vi "Process Laser State.vi"(7 "error in (no error)":errorcluster, 9 "Data":string, 10 "object in":refnum<class "Laser Ethernet Cabinet.lvclass">) -> (0 "error out":errorcluster, 3 "object out":refnum<class "Laser Ethernet Cabinet.lvclass">)   [LabVIEW 2023, in "Laser Ethernet Cabinet.lvclass"]
uses:
  Laser Ethernet Cabinet.lvclass
  raw_status.ctl
  Laser Ethernet Cabinet.lvclass/Laser Ethernet Cabinet.ctl
  <vilib>/Utility/Data Type/NI_Data Type.lvlib
panel:
  in  "Raw Status":T1
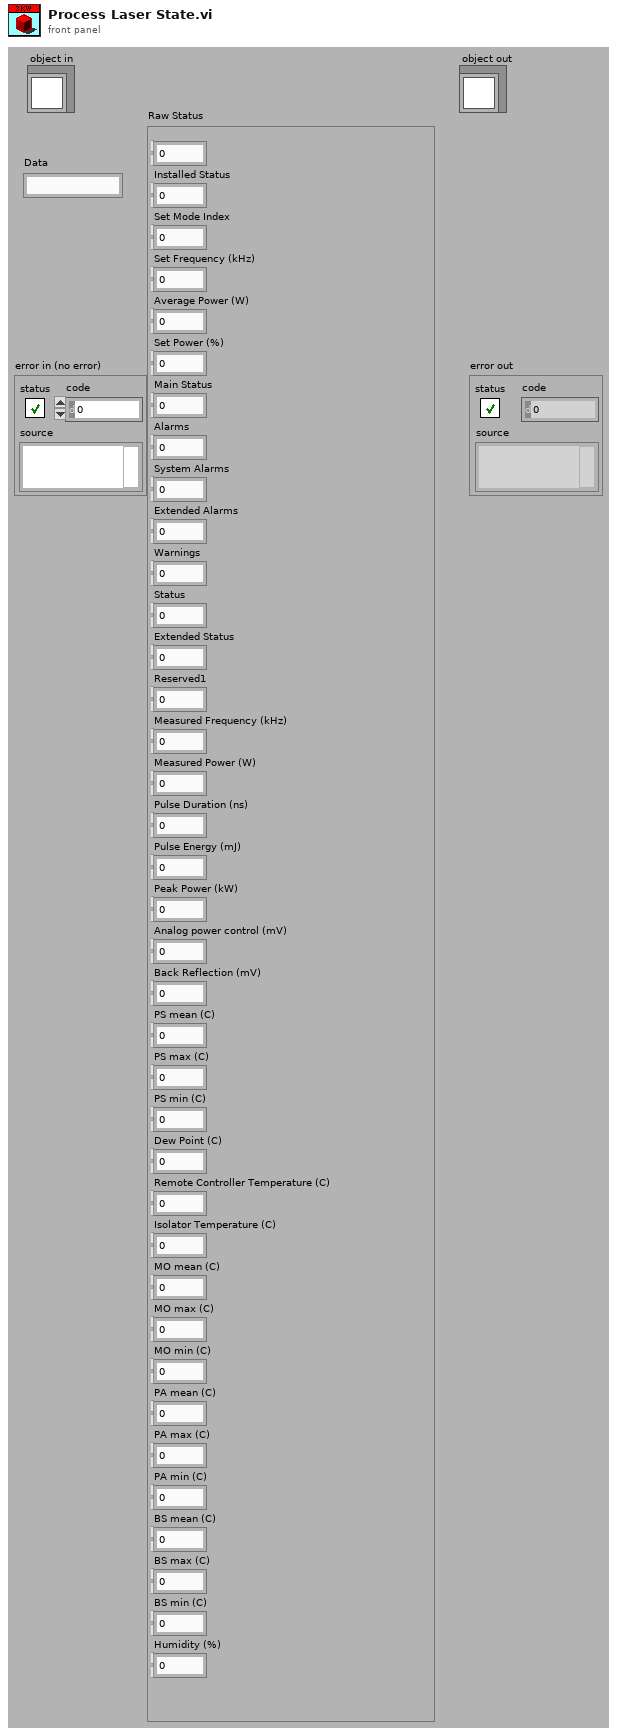
[diagram p1: front panel]
types:
  T1 = typedef "Laser Ethernet Cabinet.lvclass/raw_status.ctl" = cluster{"Version":u16, "Installed Status":u32, "Set Mode Index":u16, "Set Frequency (kHz)":sgl, "Average Power (W)":sgl, "Set Power (%)":sgl, "Main Status":u32, "Alarms":u32, "System Alarms":u32, "Extended Alarms":u32, "Warnings":u32, "Status":u32, "Extended Status":u32, "Reserved1":u16, "Measured Frequency (kHz)":sgl, "Measured Power (W)":sgl, "Pulse Duration (ns)":u32, "Pulse Energy (mJ)":sgl, "Peak Power (kW)":sgl, "Analog power control (mV)":sgl, "Back Reflection (mV)":sgl, "PS mean (C)":sgl, "PS max (C)":sgl, "PS min (C)":sgl, "Dew Point (C)":sgl, "Remote Controller Temperature (C)":sgl, "Isolator Temperature (C)":sgl, "MO mean (C)":sgl, "MO max (C)":sgl, "MO min (C)":sgl, "PA mean (C)":sgl, "PA max (C)":sgl, "PA min (C)":sgl, "BS mean (C)":sgl, "BS max (C)":sgl, "BS min (C)":sgl, "Humidity (%)":sgl}
  T2 = typedef "NI_Data Type.lvlib/Data Type.ctl" = enum8{"Invalid Type", "Void", "I8", "I16", "I32", "I64", "U8", "U16", "U32", "U64", "Single Float", "Double Float", "Extended Float", "Single Complex", "Double Complex", "Extended Complex", "Enum U8", "Enum U16", "Enum U32", "Enum U64", "Single Float With Unit", "Double Float With Unit", "Extended Float With Unit", "Single Complex with Unit", "Double Complex with Unit", "Extended Complex with Unit", "Boolean", "String", "Path", "Picture", "Tag", "Array", "Cluster", "Variant", "LV Variant", "Waveform", "Timestamp", "Digital Waveform", "Digital Data", "ExpressData", "Refnum", "External Data", "VI", "Poly VI", "LabVIEW Class Instance", "Fixed Point", "Set Collection", "Map Collection"}
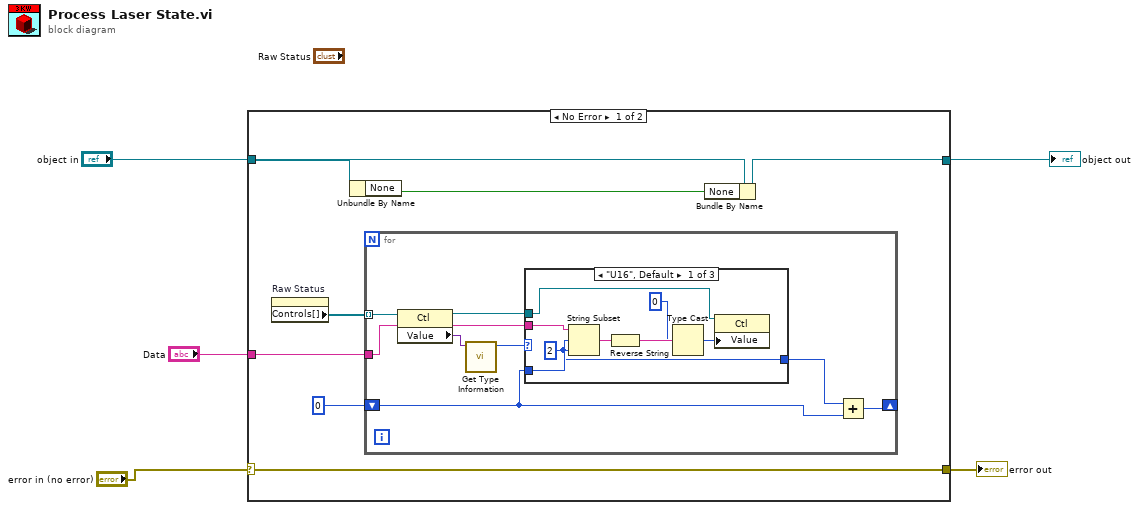
[diagram p0: block diagram]
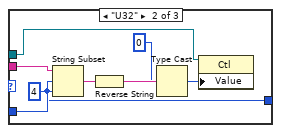
[diagram p2: hidden frame]
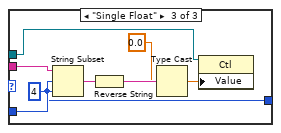
[diagram p3: hidden frame]
diagram:
  n1 = case shown="No Error" "error in (no error)" {
    selector: "error in (no error)" -> [w11 w46]
    tunnel: [w11 w46] -> w1
    tunnel: [w9 w45] -> w2
    tunnel: "object in" -> [w10 w45]
    tunnel: "Data" -> [w7 _]
    frame No Error {
      n2 = property on="Raw Status" class="Clust (strict)"() -> ("Controls[]"=w8:refnum<vi>[])  [unwired: 2 in, 2 out]
      n3 = Unbundle By Name(w10) -> ("None"=w12:bool)
      n4 = for {
        tunnel: w8 -> [w17] mode=indexing
        tunnel: w7 -> [w16]
        shift-right: [w13] -> _
        shift-left: 0 ("offset (0)") -> [w14]
        n5 = property class="Ctl"(reference=w17) -> (reference out=w19:refnum<vi>, "Value"=w20:variant)  [unwired: 1 in, 1 out]
        n6 = call <vilib>:"Get Type Information.vi"("variant"=w20) -> ("type"=w18:T2)  [unwired: 6 in, 4 out]
        n7 = case shown="\"U16\", Default" w18 {
          tunnel: w16 -> [w24 w32 w40]
          tunnel: w19 -> [w25 w34 w42]
          tunnel: w14 -> [w22 w30 w38]
          tunnel: [w21 w29 w37] -> w15
          frame "U16", Default {
            w21 = 2
            n8 = String Subset(string=w24, offset (0)=w22, length (rest)=w21) -> (substring=w23:string)
            n9 = Reverse String(1:w23) -> (0:w28:string)
            n10 = Type Cast(type=u16 0, x=w28) -> (*(type *) &x=w26:u16)
            n11 = property class="Ctl"(reference=w25, "Value"=w26) -> ()  [unwired: 1 in, 2 out]
          }
          frame "U32" {
            w29 = 4
            n12 = String Subset(string=w32, offset (0)=w30, length (rest)=w29) -> (substring=w31:string)
            n13 = Reverse String(1:w31) -> (0:w36:string)
            n14 = Type Cast(type=u32 0, x=w36) -> (*(type *) &x=w33:u32)
            n15 = property class="Ctl"(reference=w34, "Value"=w33) -> ()  [unwired: 1 in, 2 out]
          }
          frame "Single Float" {
            w37 = 4
            n16 = String Subset(string=w40, offset (0)=w38, length (rest)=w37) -> (substring=w39:string)
            n17 = Reverse String(1:w39) -> (0:w44:string)
            n18 = Type Cast(type=sgl 0.0, x=w44) -> (*(type *) &x=w41:sgl)
            n19 = property class="Ctl"(reference=w42, "Value"=w41) -> ()  [unwired: 1 in, 2 out]
          }
        }
        n20 = Add(x=w15, y=w14) -> (x+y=w13:i32)
      }
      n21 = Bundle By Name(cluster=w10, "None"=w12) -> (w9:refnum<class "Laser Ethernet Cabinet.lvclass">)
    }
    frame Error {
    }
  }
  "error out" <- w1
  "object out" <- w2
